vi "ATS_StartAcquisition.vi"(8 "error in (no error)":errorcluster, 11 "Handle In":u32) -> (0 "error out":errorcluster, 3 "Handle out":u32)   [LabVIEW 2016]
panel:
  out "Return Code":u32
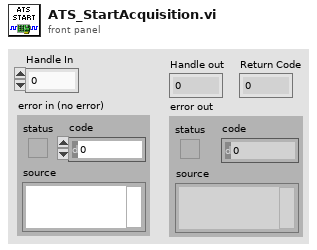
[diagram p1: front panel]
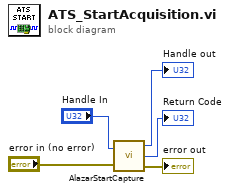
[diagram p0: block diagram]
diagram:
  n1 = call "AlazarStartCapture.vi"("Handle"="Handle In", "error in (no error)"="error in (no error)") -> ("Handle"=→"Handle out":u32, "Return Code"=→"Return Code":u32, "error out"=→"error out":errorcluster)
